vi "GetMessage.vi"(8 "error in":errorcluster, 9 "Amout":string, 10 "Account":T1, 11 "Message Type":string) -> (0 "error out":errorcluster, 3 "Message":string)   [LabVIEW 2016]
doc: "Return message in function of the message type\nAnd replace AMOUNT, NAME field in message"
uses:
  Controls/Account.ctl
  Controls/Message.ctl
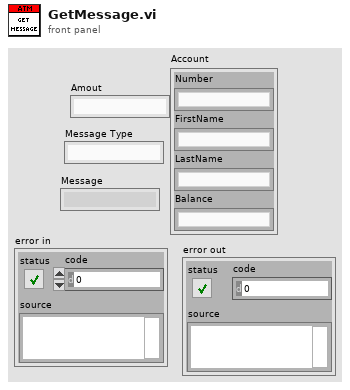
[diagram p1: front panel]
types:
  T1 = typedef "Account.ctl" = cluster{"Number":string, "FirstName":string, "LastName":string, "Balance":string}
  T2 = typedef "Message.ctl" = string[][]
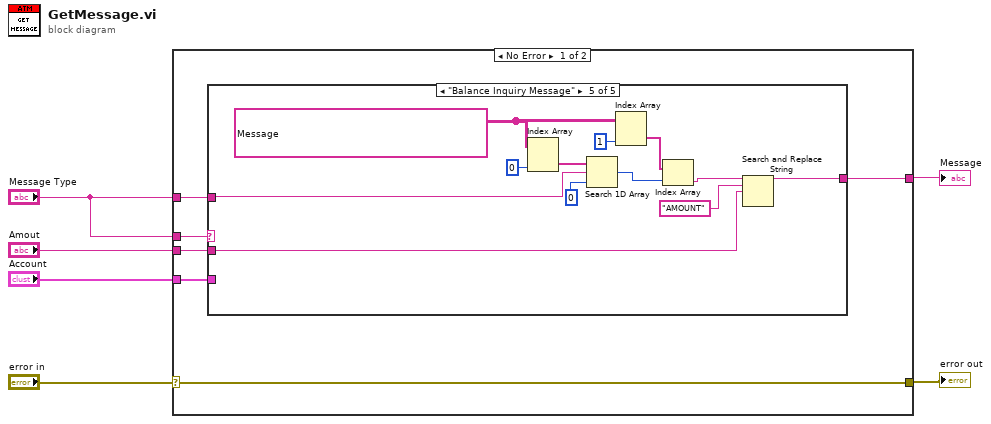
[diagram p0: block diagram]
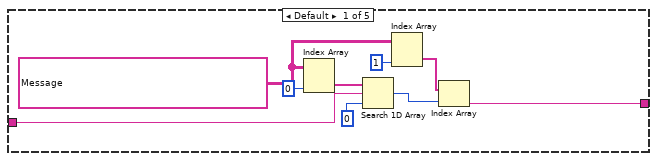
[diagram p2: hidden frame]
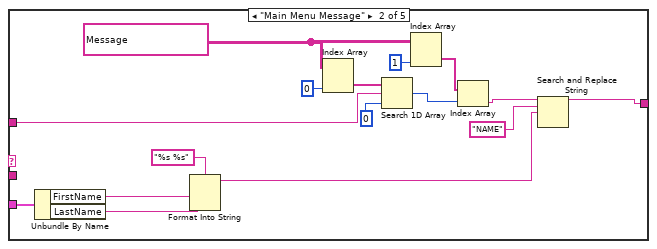
[diagram p3: hidden frame]
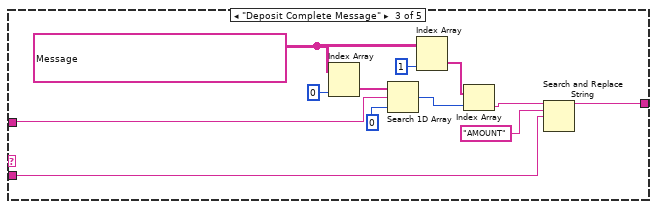
[diagram p4: hidden frame]
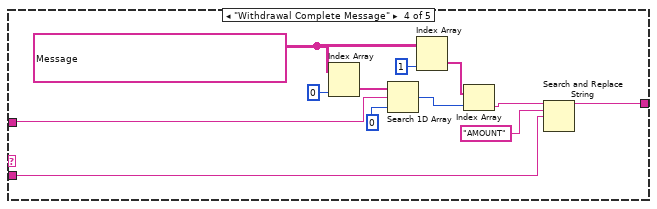
[diagram p5: hidden frame]
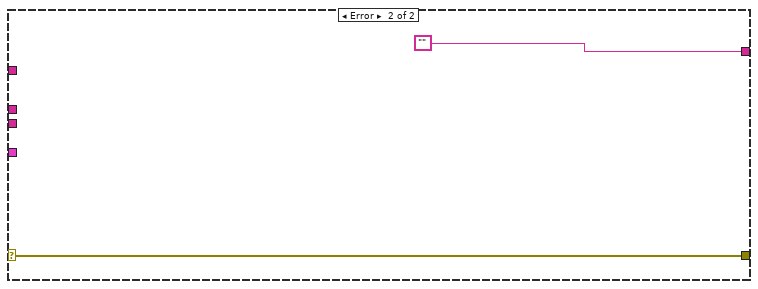
[diagram p6: hidden frame]
diagram:
  n1 = case shown="No Error" "error in" {
    selector: "error in" -> [w10 w75]
    tunnel: "Message Type" -> [w12 _]
    tunnel: [w11 ""] -> w6
    tunnel: [w10 w75] -> w4
    tunnel: "Message Type" -> [w9 _]
    tunnel: "Account" -> [w8 _]
    tunnel: "Amout" -> [w7 _]
    frame No Error {
      n2 = case shown="\"Balance Inquiry Message\"" w9 {
        tunnel: w12 -> [w14 w31 w40 w52 w64]
        tunnel: [w15 w23 w39 w51 w63] -> w11
        tunnel: w8 -> [_ w29 _ _ _]
        tunnel: w7 -> [_ _ w38 w50 w62]
        frame Default {
          w13 = T2 [["Welcome Message", "Welcome to Acme Bank. \nPlease insert your card \nand enter your account \nnumber in the User Input. \n \nPress Enter (E) when done."], ["Main Menu Message", "Welcome to Acme Bank \nNAME\n \nPlease select transaction \nby using the buttons."], ["Account Verification Failed Message", "Account Information Incorrect \nPlease Re-Enter Account Number. \nPress Enter (E) when done"], ["Session Terminate Message", "Your session has been terminated \ndue to inactivity or menu selection. \nPlease take your card \n \nGoodbye!"], ["Deposit Message", "Please enter amount to deposit and press \nEnter (E) when done"], ["Deposit Complete Message", "$ AMOUNT Deposited"], ["Withdrawal Message", "Please enter amount to withdraw and press \nEnter (E) when done"], ["Withdrawal Complete Message", "$ AMOUNT Withdrawn"], ["Withdrawal Failed Message", "Insufficient funds in account \nPlease check your balance \nand try again"], ["Balance Inquiry Message", "Your Balance Is: \n$ AMOUNT"]] ("Array")
          n3 = Index Array(array=w13, index (col)=0 ("disabled index (col)")) -> (element=w17:string[])  [unwired: 1 in]
          n4 = Search 1D Array(1D array=w17, element=w14, start index (0)=0) -> (index of element=w19:i32)
          n5 = Index Array(array=w13, index (col)=1 ("disabled index (col)")) -> (element=w21:string[])  [unwired: 1 in]
          n6 = Index Array(array=w21, index=w19) -> (element=w15:string)
        }
        frame "Main Menu Message" {
          w22 = T2 [["Welcome Message", "Welcome to Acme Bank. \nPlease insert your card \nand enter your account \nnumber in the User Input. \n \nPress Enter (E) when done."], ["Main Menu Message", "Welcome to Acme Bank \nNAME\n \nPlease select transaction \nby using the buttons."], ["Account Verification Failed Message", "Account Information Incorrect \nPlease Re-Enter Account Number. \nPress Enter (E) when done"], ["Session Terminate Message", "Your session has been terminated \ndue to inactivity or menu selection. \nPlease take your card \n \nGoodbye!"], ["Deposit Message", "Please enter amount to deposit and press \nEnter (E) when done"], ["Deposit Complete Message", "$ AMOUNT Deposited"], ["Withdrawal Message", "Please enter amount to withdraw and press \nEnter (E) when done"], ["Withdrawal Complete Message", "$ AMOUNT Withdrawn"], ["Withdrawal Failed Message", "Insufficient funds in account \nPlease check your balance \nand try again"], ["Balance Inquiry Message", "Your Balance Is: \n$ (Balance Amount from file)"]] ("Array")
          n7 = Unbundle By Name(w29) -> ("FirstName"=w28:string, "LastName"=w27:string)
          n8 = Format Into String(format string="%s %s", w28, w27) -> (resulting string=w24:string)  [unwired: 2 in, 1 out]
          n9 = Index Array(array=w22, index (col)=0 ("disabled index (col)")) -> (element=w36:string[])  [unwired: 1 in]
          n10 = Search 1D Array(1D array=w36, element=w31, start index (0)=0) -> (index of element=w34:i32)
          n11 = Index Array(array=w22, index (col)=1 ("disabled index (col)")) -> (element=w32:string[])  [unwired: 1 in]
          n12 = Index Array(array=w32, index=w34) -> (element=w26:string)
          n13 = Search and Replace String(input string=w26, search string="NAME", replace string=w24) -> (result string=w23:string)  [unwired: 5 in, 3 out]
        }
        frame "Deposit Complete Message" {
          w41 = T2 [["Welcome Message", "Welcome to Acme Bank. \nPlease insert your card \nand enter your account \nnumber in the User Input. \n \nPress Enter (E) when done."], ["Main Menu Message", "Welcome to Acme Bank \nNAME\n \nPlease select transaction \nby using the buttons."], ["Account Verification Failed Message", "Account Information Incorrect \nPlease Re-Enter Account Number. \nPress Enter (E) when done"], ["Session Terminate Message", "Your session has been terminated \ndue to inactivity or menu selection. \nPlease take your card \n \nGoodbye!"], ["Deposit Message", "Please enter amount to deposit and press \nEnter (E) when done"], ["Deposit Complete Message", "$ AMOUNT Deposited"], ["Withdrawal Message", "Please enter amount to withdraw and press \nEnter (E) when done"], ["Withdrawal Complete Message", "$ AMOUNT Withdrawn"], ["Withdrawal Failed Message", "Insufficient funds in account \nPlease check your balance \nand try again"], ["Balance Inquiry Message", "Your Balance Is: \n$ (Balance Amount from file)"]] ("Array")
          n14 = Index Array(array=w41, index (col)=0 ("disabled index (col)")) -> (element=w48:string[])  [unwired: 1 in]
          n15 = Search 1D Array(1D array=w48, element=w40, start index (0)=0) -> (index of element=w46:i32)
          n16 = Index Array(array=w41, index (col)=1 ("disabled index (col)")) -> (element=w44:string[])  [unwired: 1 in]
          n17 = Index Array(array=w44, index=w46) -> (element=w43:string)
          n18 = Search and Replace String(input string=w43, search string="AMOUNT", replace string=w38) -> (result string=w39:string)  [unwired: 5 in, 3 out]
        }
        frame "Withdrawal Complete Message" {
          w53 = T2 [["Welcome Message", "Welcome to Acme Bank. \nPlease insert your card \nand enter your account \nnumber in the User Input. \n \nPress Enter (E) when done."], ["Main Menu Message", "Welcome to Acme Bank \nNAME\n \nPlease select transaction \nby using the buttons."], ["Account Verification Failed Message", "Account Information Incorrect \nPlease Re-Enter Account Number. \nPress Enter (E) when done"], ["Session Terminate Message", "Your session has been terminated \ndue to inactivity or menu selection. \nPlease take your card \n \nGoodbye!"], ["Deposit Message", "Please enter amount to deposit and press \nEnter (E) when done"], ["Deposit Complete Message", "$ AMOUNT Deposited"], ["Withdrawal Message", "Please enter amount to withdraw and press \nEnter (E) when done"], ["Withdrawal Complete Message", "$ AMOUNT Withdrawn"], ["Withdrawal Failed Message", "Insufficient funds in account \nPlease check your balance \nand try again"], ["Balance Inquiry Message", "Your Balance Is: \n$ (Balance Amount from file)"]] ("Array")
          n19 = Index Array(array=w53, index (col)=0 ("disabled index (col)")) -> (element=w60:string[])  [unwired: 1 in]
          n20 = Search 1D Array(1D array=w60, element=w52, start index (0)=0) -> (index of element=w58:i32)
          n21 = Index Array(array=w53, index (col)=1 ("disabled index (col)")) -> (element=w56:string[])  [unwired: 1 in]
          n22 = Index Array(array=w56, index=w58) -> (element=w55:string)
          n23 = Search and Replace String(input string=w55, search string="AMOUNT", replace string=w50) -> (result string=w51:string)  [unwired: 5 in, 3 out]
        }
        frame "Balance Inquiry Message" {
          w65 = T2 [["Welcome Message", "Welcome to Acme Bank. \nPlease insert your card \nand enter your account \nnumber in the User Input. \n \nPress Enter (E) when done."], ["Main Menu Message", "Welcome to Acme Bank \nNAME\n \nPlease select transaction \nby using the buttons."], ["Account Verification Failed Message", "Account Information Incorrect \nPlease Re-Enter Account Number. \nPress Enter (E) when done"], ["Session Terminate Message", "Your session has been terminated \ndue to inactivity or menu selection. \nPlease take your card \n \nGoodbye!"], ["Deposit Message", "Please enter amount to deposit and press \nEnter (E) when done"], ["Deposit Complete Message", "$ AMOUNT Deposited"], ["Withdrawal Message", "Please enter amount to withdraw and press \nEnter (E) when done"], ["Withdrawal Complete Message", "$ AMOUNT Withdrawn"], ["Withdrawal Failed Message", "Insufficient funds in account \nPlease check your balance \nand try again"], ["Balance Inquiry Message", "Your Balance Is: \n$ AMOUNT"]] ("Array")
          n24 = Index Array(array=w65, index (col)=0 ("disabled index (col)")) -> (element=w72:string[])  [unwired: 1 in]
          n25 = Search 1D Array(1D array=w72, element=w64, start index (0)=0) -> (index of element=w70:i32)
          n26 = Index Array(array=w65, index (col)=1 ("disabled index (col)")) -> (element=w68:string[])  [unwired: 1 in]
          n27 = Index Array(array=w68, index=w70) -> (element=w67:string)
          n28 = Search and Replace String(input string=w67, search string="AMOUNT", replace string=w62) -> (result string=w63:string)  [unwired: 5 in, 3 out]
        }
      }
    }
    frame Error {
    }
  }
  "Message" <- w6
  "error out" <- w4
